vi "Main.vi"() -> ()   [LabVIEW 2018, in "Flightweight Pattern Demo.lvclass"]
uses:
  Flightweight Pattern Demo.lvclass
  ShapeFactory Class/fwShapeFactory.lvclass
  ConsoleOut/Print Options.ctl
  Flightweight Pattern Demo.lvclass/Flightweight Pattern Demo.ctl
  Circle Class/fwCircle.lvclass/fwCircle.ctl
  Circle Class/fwCircle.lvclass
panel:
  out "error out":errorcluster
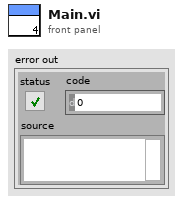
[diagram p1: front panel]
types:
  T1 = typedef "Print Options.ctl" = enum16{"Create", "Get Reference", "Print", "Print Header", "Close"}
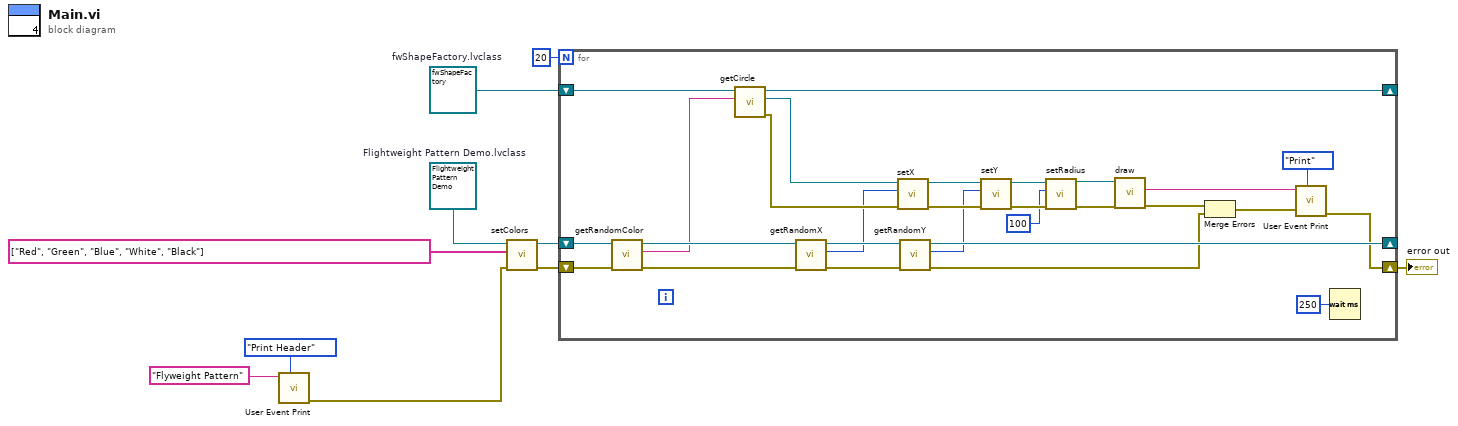
[diagram p0: block diagram]
diagram:
  w5 = refnum<class "fwShapeFactory.lvclass"> refnum  # fwShapeFactory.lvclass
  w9 = refnum<class "Flightweight Pattern Demo.lvclass"> refnum  # Flightweight Pattern Demo.lvclass
  n1 = call "User Event Print.vi"("Options"=Print_Options."Print Header", "String to Print"="Flyweight Pattern") -> ("error out"=w2:errorcluster)  [unwired: 8 in, 1 out]
  n2 = call "setColors.vi"("error in (no error)"=w2, "colors"=string[] ["Red", "Green", "Blue", "White", "Black"], "Flightweight Pattern Demo in"=w9) -> ("error out"=w6:errorcluster, "Flightweight Pattern Demo out"=w7:refnum<class "Flightweight Pattern Demo.lvclass">)  [unwired: 7 in]
  n3 = for {
    N: 20 -> [_]
    shift-right: [w34] -> _
    shift-left: w7 -> [w38]
    shift-right: [w18] -> _
    shift-left: w5 -> [w17]
    shift-right: [w11] -> w1
    shift-left: w6 -> [w27]
    n4 = call "getRandomColor.vi"("error in (no error)"=w27, "Flightweight Pattern Demo in"=w38) -> ("error out"=w16:errorcluster, "Color"=w36:string, "Flightweight Pattern Demo out"=w37:refnum<class "Flightweight Pattern Demo.lvclass">)  [unwired: 7 in]
    n5 = call "getCircle.vi"("color"=w36, "fwShapeFactory in"=w17) -> ("error out"=w33:errorcluster, "fwCircle.lvclass"=w32:refnum<class "fwCircle.lvclass">, "fwShapeFactory out"=w18:refnum<class "fwShapeFactory.lvclass">)  [unwired: 7 in]
    n6 = call "getRandomX.vi"("error in (no error)"=w16, "Flightweight Pattern Demo in"=w37) -> ("error out"=w26:errorcluster, "X"=w25:i32, "Flightweight Pattern Demo out"=w35:refnum<class "Flightweight Pattern Demo.lvclass">)  [unwired: 7 in]
    n7 = call "setX.vi"("error in (no error)"=w33, "x"=w25, "fwCircle in"=w32) -> ("error out"=w31:errorcluster, "fwCircle out"=w30:refnum<class "fwCircle.lvclass">)  [unwired: 7 in]
    n8 = call "getRandomY.vi"("error in (no error)"=w26, "Flightweight Pattern Demo in"=w35) -> ("error out"=w12:errorcluster, "Y"=w24:i32, "Flightweight Pattern Demo out"=w34:refnum<class "Flightweight Pattern Demo.lvclass">)  [unwired: 7 in]
    n9 = call "setY.vi"("error in (no error)"=w31, "y"=w24, "fwCircle in"=w30) -> ("error out"=w29:errorcluster, "fwCircle out"=w28:refnum<class "fwCircle.lvclass">)  [unwired: 7 in]
    n10 = call "setRadius.vi"("error in (no error)"=w29, "radius"=100, "fwCircle in"=w28) -> ("error out"=w21:errorcluster, "fwCircle out"=w22:refnum<class "fwCircle.lvclass">)  [unwired: 7 in]
    n11 = call-dynamic "draw.vi"("error in (no error)"=w21, "fwCircle in"=w22) -> ("error out"=w14:errorcluster, "Output"=w20:string)  [unwired: 7 in, 1 out]
    n12 = Merge Errors(w14, w12) -> (w13:errorcluster)
    n13 = call "User Event Print.vi"("Options"=Print_Options."Print", "error in (no error)"=w13, "String to Print"=w20) -> ("error out"=w11:errorcluster)  [unwired: 7 in, 1 out]
    n14 = Wait (ms)(milliseconds to wait=u32 250) -> ()  [unwired: 1 out]
  }
  "error out" <- w1
